vi "Vision Research Phantom Series PhCon PhSetDllsLogOption.vi"(1 "Value":u32, 3 "SelectCode":T1=100 items=["SDLO_PHANTOM"=100, "SDLO_PHCON"=101, "SDLO_PHINT"=102, "SDLO_PHFILE"=103, "SDLO_PHSIG"=104, "SDLO_PHSIGV"=105, "SDLO_TORAM"=106], 5 "Error In (no error)":errorcluster) -> (19 "Error Out":errorcluster)   [LabVIEW 2013, in "VRI.lvlib"]
doc: "PhCon.dll \n\nPhSetDllsLogOption\nHRESULT PhSetDllsLogOption(UINT, SelectCode, UINT Value);\n\nParameters Description \nSelectCode Select the module to set the log options. Use the constants defined in PhCon.h:\n SDLO_PHANTOM\n SDLO_PHCON\n SDLO_PHINT\n SDLO_PHFILE\n SDLO_PHSIG\n SDLO_PHSIGV\n SDLO_TORAM\n to select a certain module or option.\nValue Usually set a value of 0xFFFFFFFF to enable all dumps from a module or 0 to \n disable all dumps. \nReturn HRESULT (0 = Ok)\nComments To enable collecting a log file in PhCon call this function with the parameters \n SDLO_PHCON, 0xFFFFFFFF. To stop collecting the log file call the function with\n the parameters SDLO_PHCON, 0. You can set these settings in the Phantom\n application Help/About/Logging or by calling this function from your application.\n These settings are stored in Windows registry and are unique for all applications\n that use PhCon.\n To get fast logging set the TORAM option to 1. If the application crashes or fails\n to unregister, the log information will be lost. To debug crashes set TORAM to 0."
uses:
  VRI.lvlib
  _Type Defs/PhCon SDLO.ctl
  Phantom DLLs/PhCon.Dll
panel:
  # "For instructions on the use of this VI, press Ctrl+H to display the help window and move the mouse over the icon, controls, and indicators"
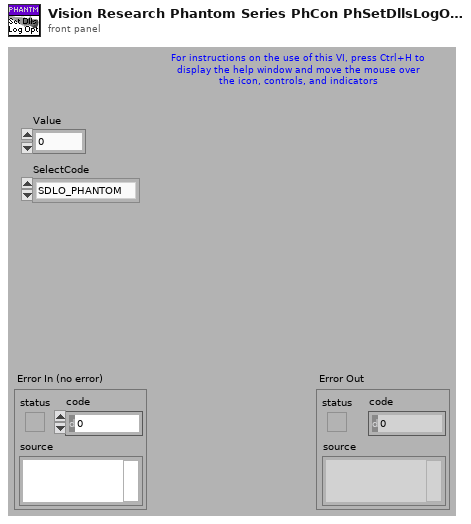
[diagram p1: front panel]
types:
  T1 = typedef "VRI.lvlib/PhCon SDLO.ctl" = u32
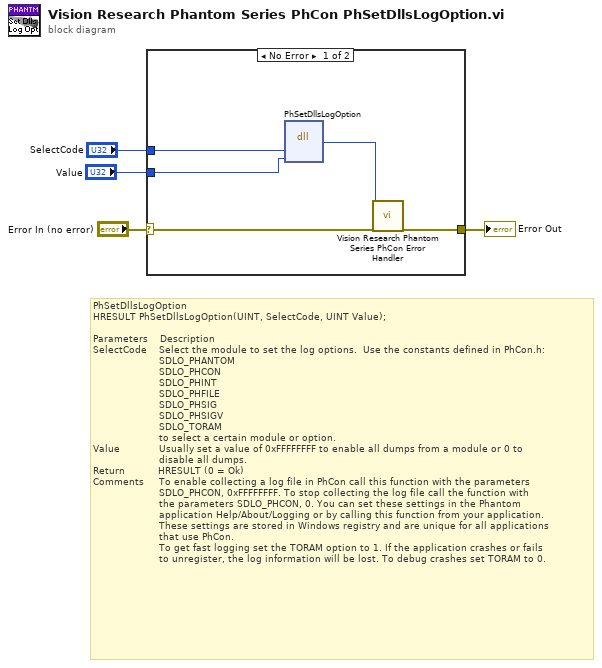
[diagram p0: block diagram]
diagram:
  # "PhSetDllsLogOption\nHRESULT PhSetDllsLogOption(UINT, SelectCode, UINT Value);\n\nParameters    Description \nSelectCode    Select the module to set the log options.  Use the constants defined in PhCon.h:\n                      SDLO_PHANTOM\n                      SDLO_PHCON\n                      SDLO_PHINT\n                      SDLO_PHFILE\n                      SDLO_PHSIG\n                      SDLO_PHSIGV\n                      SDLO_TORAM\n                      to select a certain module or option.\nValue             Usually set a value of 0xFFFFFFFF to enable all dumps from a module or 0 to \n                      disable all dumps. \nReturn           HRESULT (0 = Ok)\nComments     To enable collecting a log file in PhCon call this function with the parameters \n                      SDLO_PHCON, 0xFFFFFFFF. To stop collecting the log file call the function with\n                      the parameters SDLO_PHCON, 0. You can set these settings in the Phantom\n                      application Help/About/Logging or by calling this function from your application.\n                      These settings are stored in Windows registry and are unique for all applications\n                      that use PhCon.\n                      To get fast logging set the TORAM option to 1. If the application crashes or fails\n                      to unregister, the log information will be lost. To debug crashes set TORAM to 0."
  n1 = case shown="No Error" "Error In (no error)" {
    selector: "Error In (no error)" -> [w9 w10]
    tunnel: [w8 w10] -> w3
    tunnel: "SelectCode" -> [w7 _]
    tunnel: "Value" -> [w6 _]
    frame No Error {
      n2 = dll-call lib="C:/Projects/SDK/64-bit/Vision Research Phantom Series Labview Driver/Phantom DLLs/PhCon.dll" fn="PhSetDllsLogOption"("SelectCode"=w7, "Value"=w6) -> ("HRESULT"=w5:i32)  [unwired: 5 in, 2 out]
      n3 = call "Vision Research Phantom Series PhCon Error Handler.vi"("ErrNo"=w5, "Error In (no error)"=w9) -> ("Error Out"=w8:errorcluster)  [unwired: 17 out]
    }
    frame Error {
    }
  }
  "Error Out" <- w3
